vi "Car Wash System.vi"() -> ()   [LabVIEW 2024]
uses:
  ctl/Options Indicator.ctl
  ctl/Wash Options in.ctl
  ctl/State Machine.ctl
  ctl/Login State Machine.ctl
  <vilib>/Utility/file.llb/Write Delimited Spreadsheet (string).vi
  <vilib>/Utility/file.llb/Read Delimited Spreadsheet (string).vi
panel:
  in  "stop":bool
  in  "Options":T1
  in  "Start Button":bool
  out "Car Wash Indicator":T2
  out "Wash Vacant":bool
  out "Elapsed Time":dbl format="%#_3g"
  in  "Car Position Slider":u8(slide) max=3 scale=0.0..4.0
  in  "Stop Program":bool
  out "appended path":path
  out "Numeric":i32
  in  "Tab Control":enum32{"Login", "Register"}(tab)
  in  "Login":bool
  in  "Username":string
  in  "Password":string
  out "Status":bool
  in  "Username":string
  in  "Password":string
  in  "Register":bool
  out "Array":string[](array[string])
  out "error out":errorcluster
  in  "error in":errorcluster
  # "Entry Console"
  # "Car Wash Display"
  # "Wash Entry"
  # "Wash Options"
  # "Car Wash Indicator"
  # "Start"
  # "Car Position Simulation"
  # "Underbody Wash\nBug Remover"
  # "Pre-Soak\nH-P Wash\nL-P Wax\nSpot Free Rinse"
  # "Tire Shine\nAir Dry"
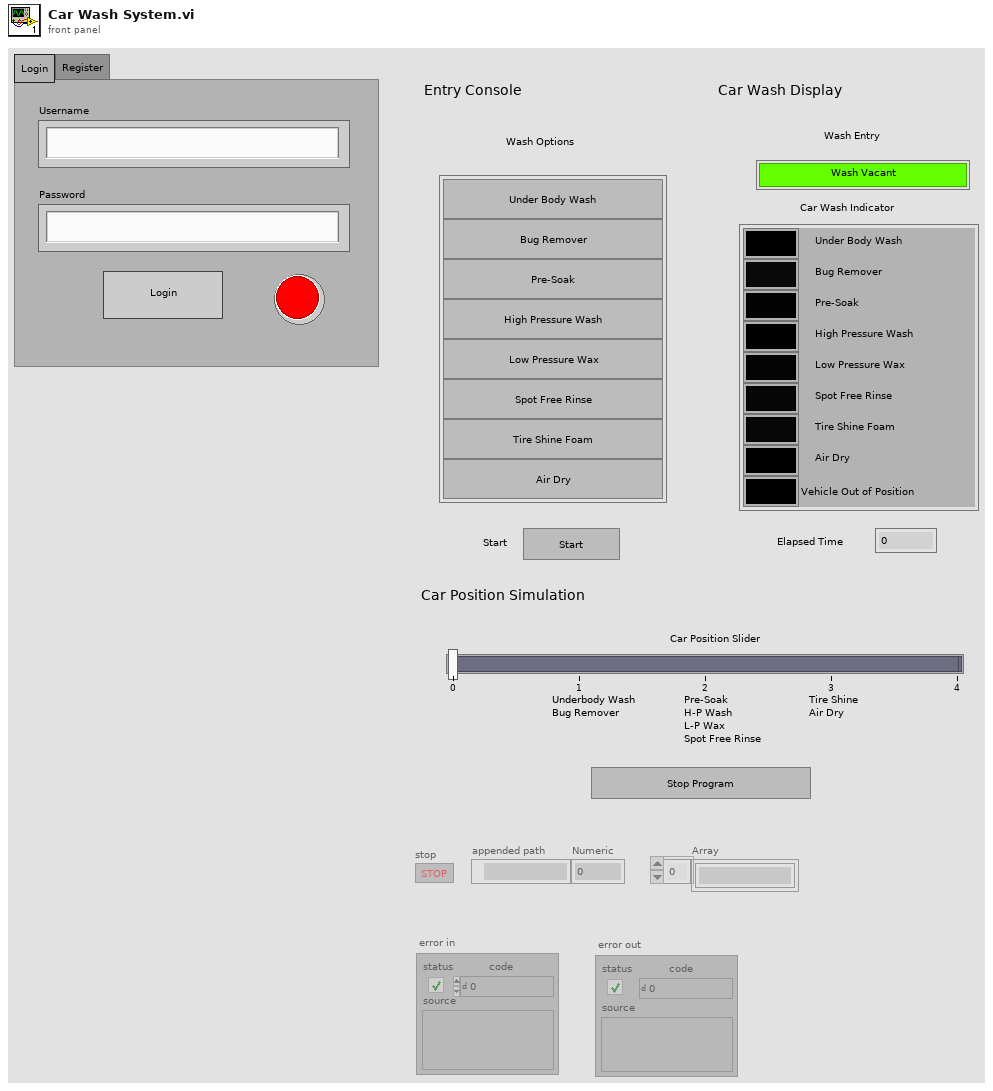
[diagram p1: front panel]
types:
  T1 = typedef "Wash Options in.ctl" = cluster{"Under Body Wash":bool, "Bug Remover":bool, "Pre-Soak":bool, "High Pressure Wash":bool, "Low Pressure Wax":bool, "Spot Free Rinse":bool, "Tire Shine Foam":bool, "Air Dry":bool}
  T2 = typedef "Options Indicator.ctl" = cluster{"Under Body Wash":bool, "Bug Remover":bool, "Pre-Soak":bool, "High Pressure Wash":bool, "Low Pressure Wax":bool, "Spot Free Rinse":bool, "Tire Shine Foam":bool, "Air Dry":bool, "Vehicle Out of Position":bool}
  T3 = typedef "Login State Machine.ctl" = enum16{"Init", "Wait", "Check", "Login", "Registration", "End"}
  T4 = typedef "State Machine.ctl" = enum16{"Initialize", "Wait", "Start", "Time", "Reset", "Stop"}
  T5 = enum8{"Enabled", "Disabled", "Disabled and Grayed Out"}
  T6 = cluster{"Under Body Wash":bool, "Bug Remover":bool, "Pre-Soak":bool, "High Pressure Wash":bool, "Low Pressure Wax":bool, "Spot Free Rinse":bool, "Tire Shine Foam":bool, "Air Dry":bool, "Vehicle Out of Position":bool}
  T7 = typedef "WashOptionsTypedef.ctl" = enum16{"Under Body Wash", "Bug Remover", "Pre-soak", "High Pressure Wash", "Low Pressure Wash", "Spot Free Rinse", "Tire Shine Foam", "Air Dry"}
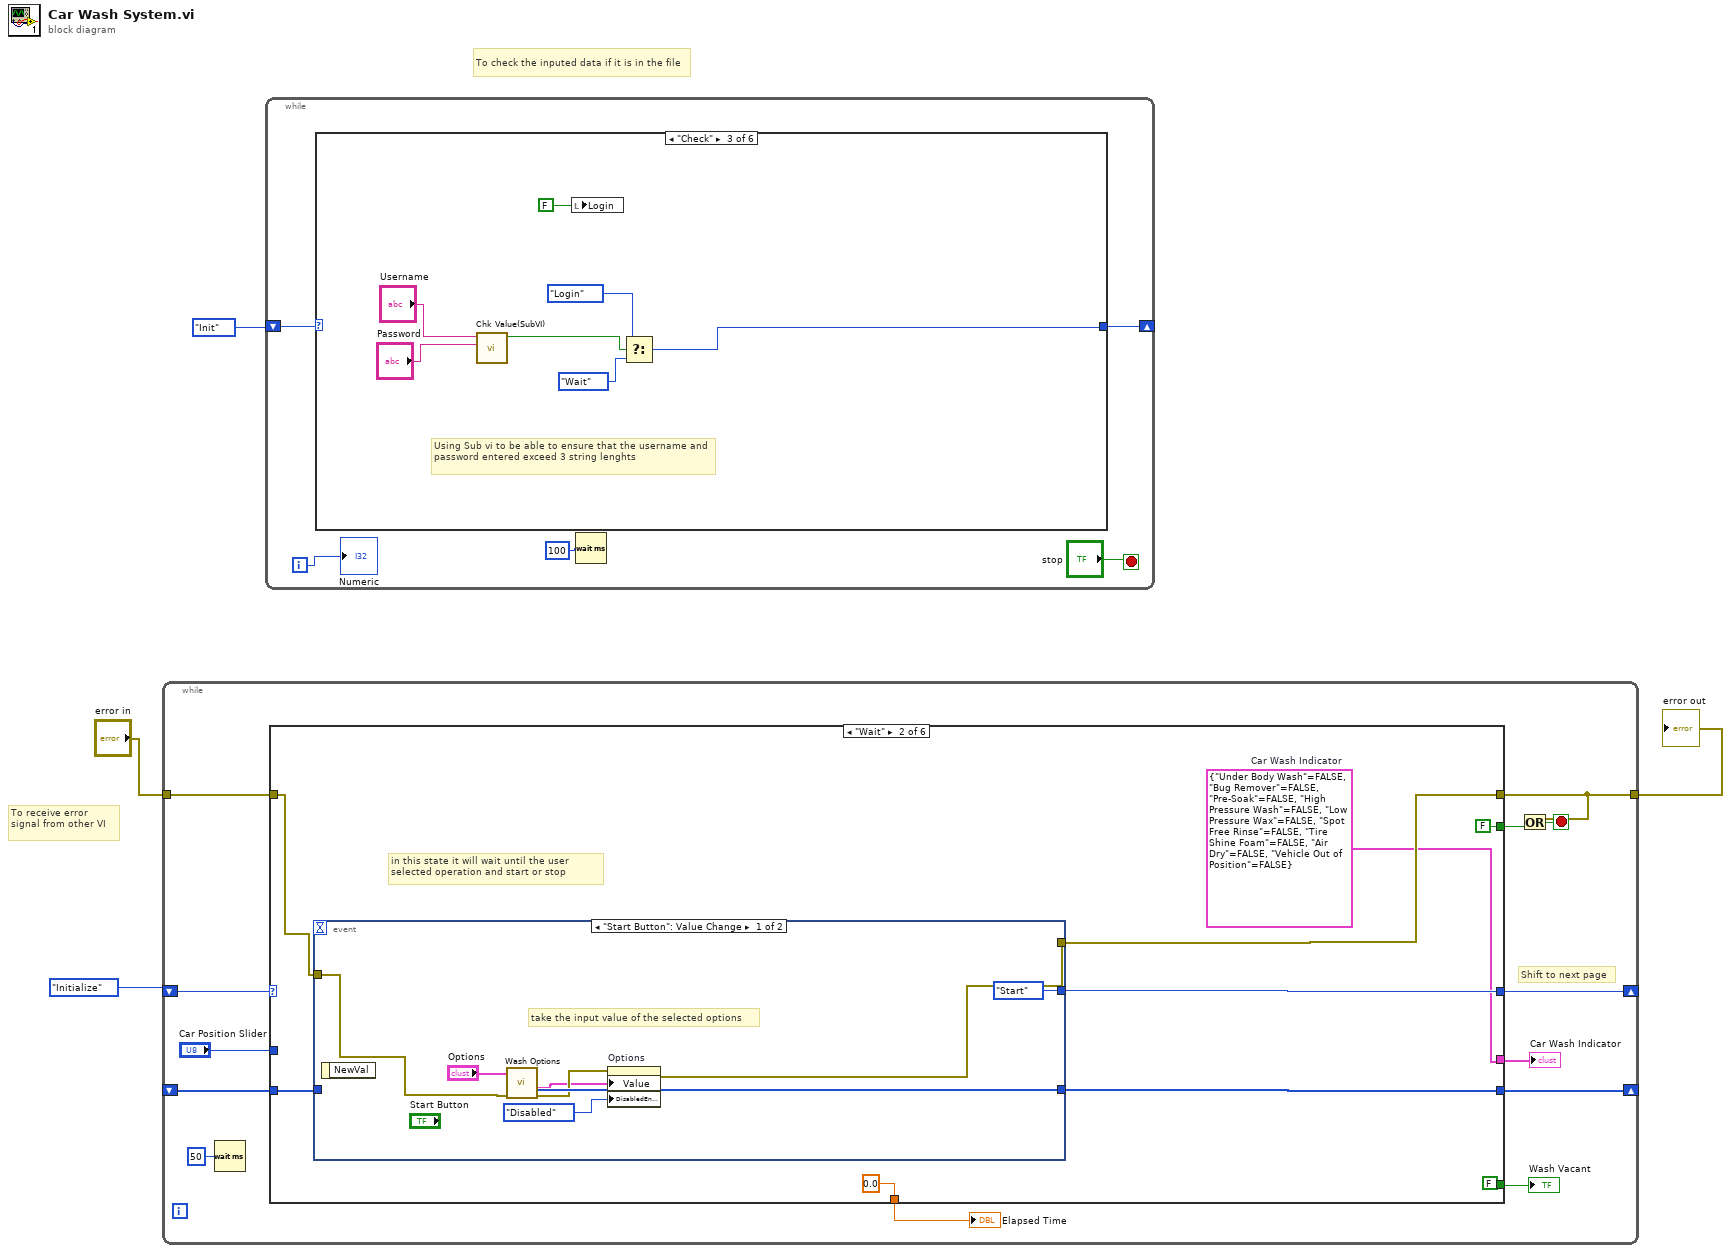
[diagram p0: block diagram]
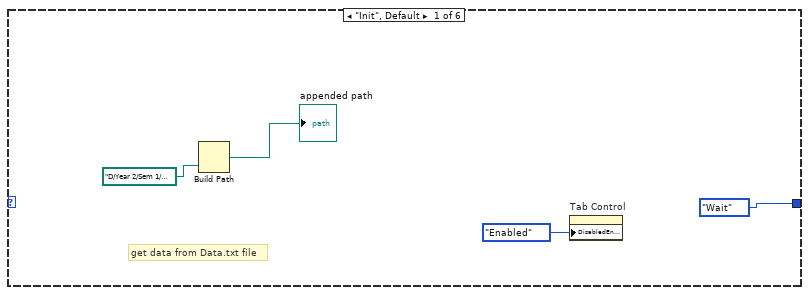
[diagram p2: hidden frame]
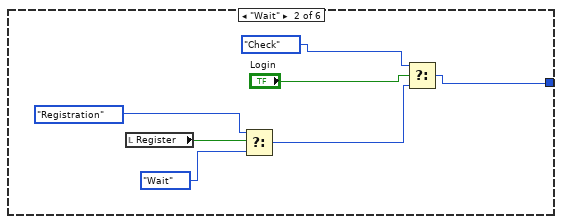
[diagram p3: hidden frame]
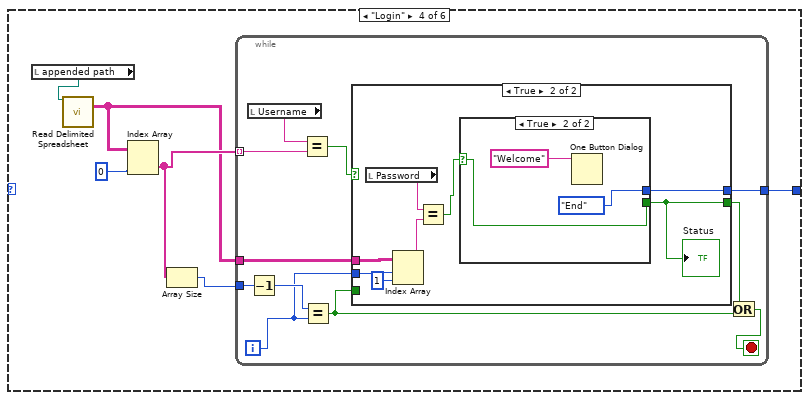
[diagram p4: hidden frame]
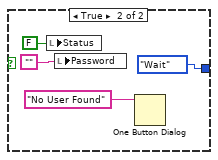
[diagram p6: hidden frame]
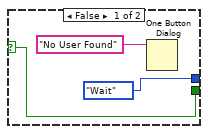
[diagram p7: hidden frame]
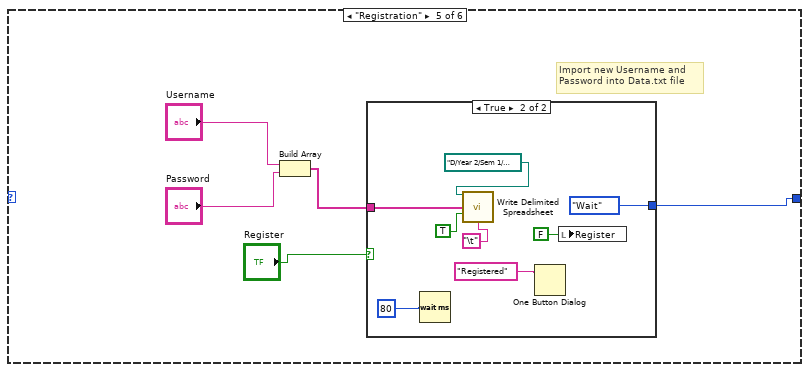
[diagram p8: hidden frame]
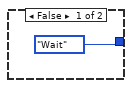
[diagram p9: hidden frame]
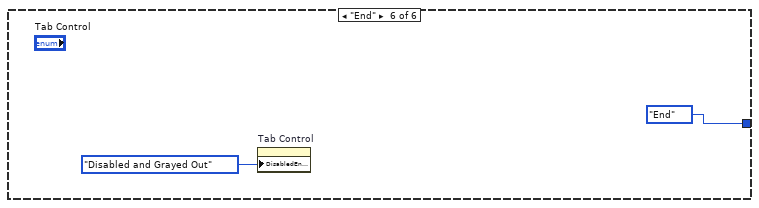
[diagram p10: hidden frame]
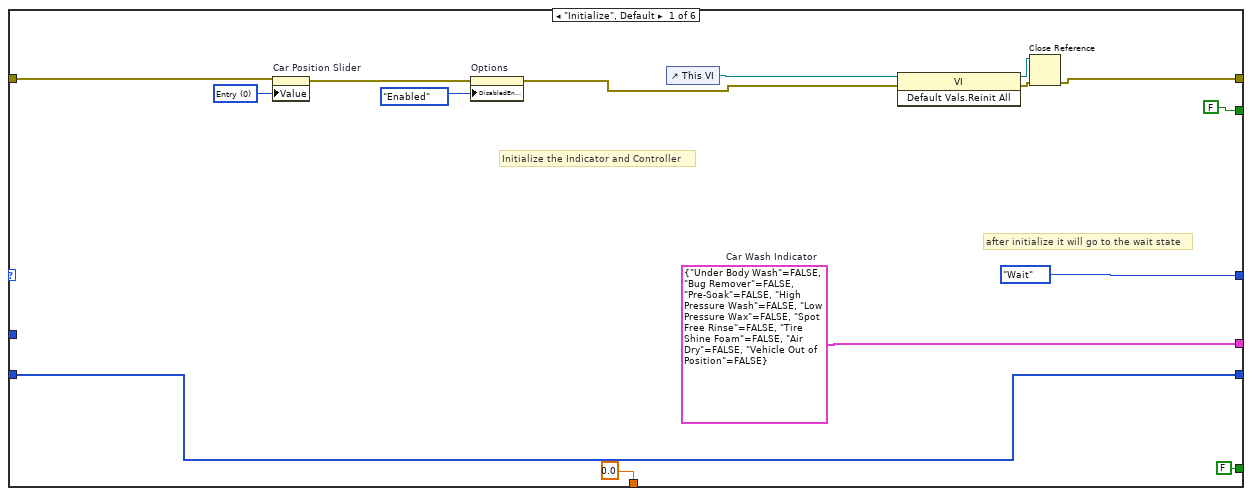
[diagram p11: hidden frame]
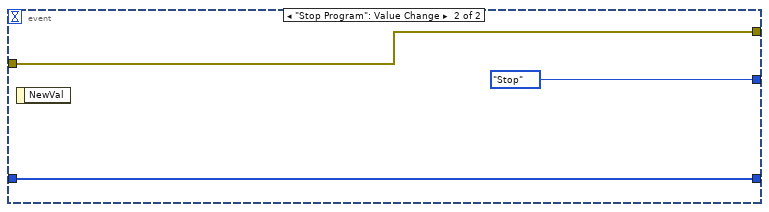
[diagram p12: hidden frame]
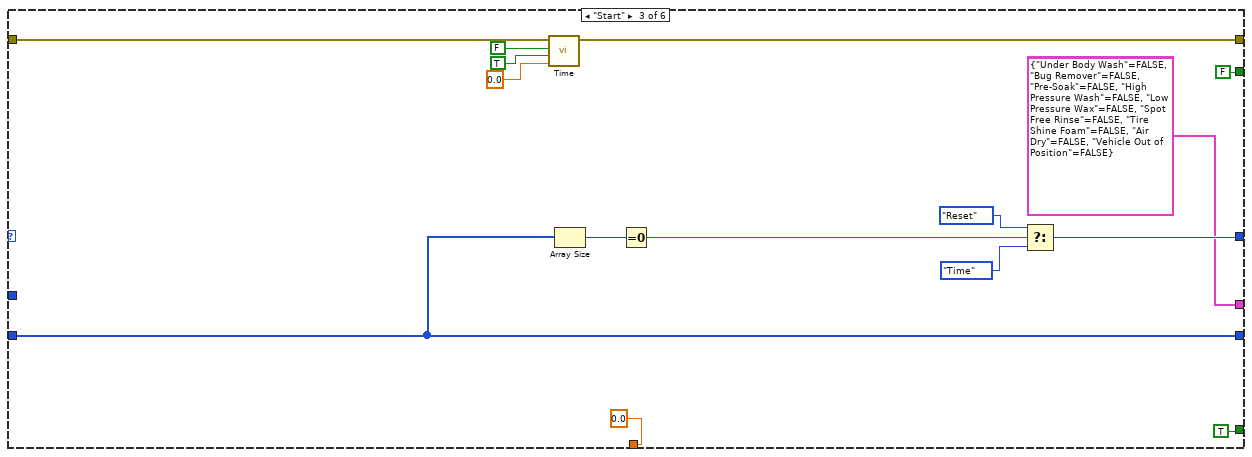
[diagram p13: hidden frame]
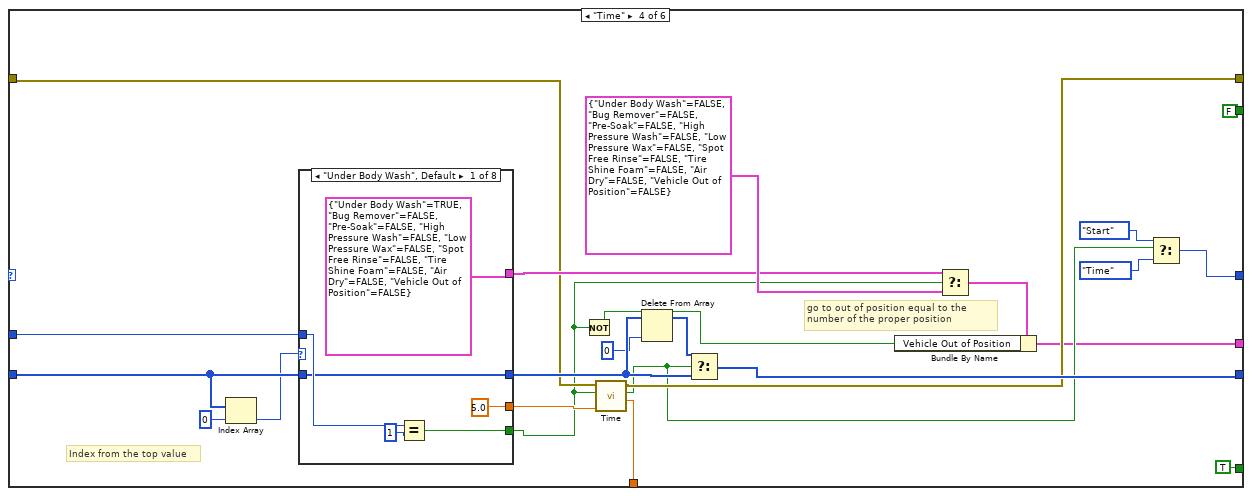
[diagram p14: hidden frame]
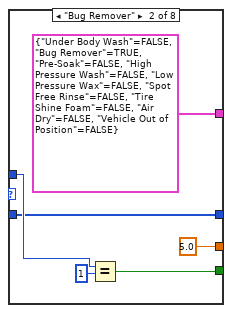
[diagram p15: hidden frame]
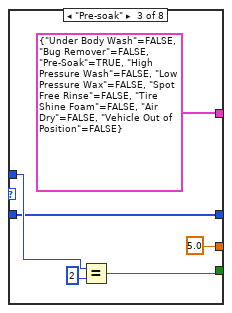
[diagram p16: hidden frame]
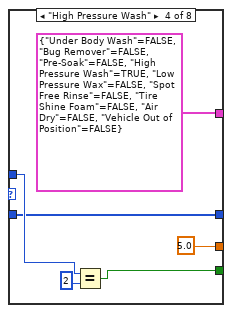
[diagram p17: hidden frame]
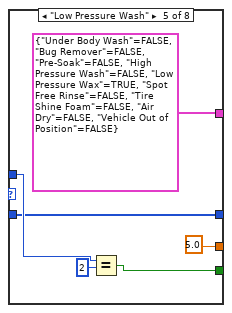
[diagram p18: hidden frame]
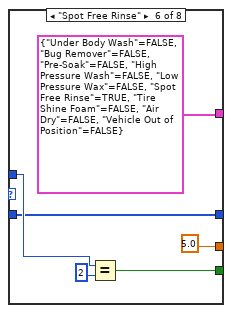
[diagram p19: hidden frame]
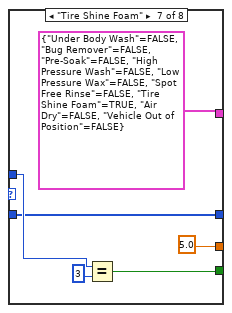
[diagram p20: hidden frame]
diagram:
  # "To check the inputed data if it is in the file"
  # "To receive error signal from other VI"
  n1 = while {
    shift-right: [w15] -> _
    shift-left: State_Machine."Initialize" -> [w16]
    shift-right: [w14] -> _
    shift-left: _ -> [w13]
    tunnel: "error in" -> [w11]
    tunnel: [w9] -> w4
    stop <- w10 stop-if-true
    # "Shift to next page"
    n2 = Wait (ms)(milliseconds to wait=u32 50) -> ()  [unwired: 1 out]
    n3 = case shown="\"Wait\"" w16 {
      tunnel: "Car Position Slider" -> [_ _ _ w89 w149 _]
      tunnel: [State_Machine."Wait" w41 w65 w76 w146 w156] -> w15
      tunnel: [w31 w40 w62 w79 w145 w170] -> w14
      tunnel: w13 -> [w31 w39 w62 w91 w145 w170]
      tunnel: w11 -> [w25 w38 w61 w75 w144 w165]
      tunnel: [w27 w37 w60 w74 w144 w164] -> w9
      tunnel: [FALSE FALSE FALSE FALSE FALSE TRUE] -> w8
      tunnel: [0.0 ("Elapsed Time") 0.0 ("Elapsed Time") 0.0 ("Elapsed Time") w70 0.0 ("Elapsed Time") 0.0 ("Elapsed Time")] -> w7
      tunnel: [FALSE ("Wash Vacant") FALSE ("Wash Vacant") TRUE ("Wash Vacant") TRUE ("Wash Vacant") TRUE ("Wash Vacant") FALSE ("Wash Vacant")] -> w6
      tunnel: [w18 w33 T6 {"Under Body Wash"=FALSE, "Bug Remover"=FALSE, "Pre-Soak"=FALSE, "High Pressure Wash"=FALSE, "Low Pressure Wax"=FALSE, "Spot Free Rinse"=FALSE, "Tire Shine Foam"=FALSE, "Air Dry"=FALSE, "Vehicle Out of Position"=FALSE} ("Car Wash Indicator") w68 w140 w157] -> w5
      frame "Initialize", Default {
        w26 = u8 0 items=["Entry", "Station 1", "Station 2", "Station 3", "Exit"] ("Car Position Slider")
        w18 = T6 {"Under Body Wash"=FALSE, "Bug Remover"=FALSE, "Pre-Soak"=FALSE, "High Pressure Wash"=FALSE, "Low Pressure Wax"=FALSE, "Spot Free Rinse"=FALSE, "Tire Shine Foam"=FALSE, "Air Dry"=FALSE, "Vehicle Out of Position"=FALSE}  # Car Wash Indicator
        # "after initialize it will go to the wait state"
        # "Initialize the Indicator and Controller"
        n4 = property on="Car Position Slider" class="Slide (strict)"(error in=w25, "Value"=w26) -> (error out=w23:errorcluster)  [unwired: 1 in, 1 out]
        n5 = property on="Options" class="Clust (strict)"(error in=w23, "DisabledEnum"=T5."Enabled" ("Disabled")) -> (error out=w22:errorcluster)  [unwired: 1 in, 1 out]
        n6 = control-ref of="This VI"() -> (w30:refnum<vi>)
        n7 = invoke class="VI" method="Default Vals.Reinit All"(reference=w30, error in=w22) -> (reference out=w28:refnum<vi>, error out=w29:errorcluster)  [unwired: 1 in, 1 out]
        n8 = Close Reference(reference=w28, error in (no error)=w29) -> (error out=w27:errorcluster)
      }
      frame "Wait" {
        w33 = T6 {"Under Body Wash"=FALSE, "Bug Remover"=FALSE, "Pre-Soak"=FALSE, "High Pressure Wash"=FALSE, "Low Pressure Wax"=FALSE, "Spot Free Rinse"=FALSE, "Tire Shine Foam"=FALSE, "Air Dry"=FALSE, "Vehicle Out of Position"=FALSE}  # Car Wash Indicator
        # "in this state it will wait until the user selected operation and start or stop"
        n9 = event shown="[0] \"Start Button\": Value Change" {
          selector: _ -> [_ _]
          dyn-events: _ -> [_ _]
          timeout: _ -> [_ _]
          tunnel: [State_Machine."Start" State_Machine."Stop"] -> w41
          tunnel: [w48 w51] -> w40
          tunnel: w39 -> [_ w51]
          tunnel: w38 -> [w45 w50]
          tunnel: [w43 w50] -> w37
          event "Start Button": Value Change {
            # "take the input value of the selected options"
            n10 = event-data() -> ()  [unwired: 1 in, 1 out]
            n11 = call "Wash Options.vi"("error in"=w45, "input"="Options") -> ("error out"=w44:errorcluster, "output"=w42:T1, "Array"=w48:T7[])  [unwired: 7 in]
            n12 = property on="Options" class="Clust (strict)"(error in=w44, "Value"=w42, "DisabledEnum"=T5."Disabled" ("Disabled")) -> (error out=w43:errorcluster)  [unwired: 1 in, 1 out]
          }
          event "Stop Program": Value Change {
            n13 = event-data() -> ()  [unwired: 1 in, 1 out]
          }
        }
      }
      frame "Start" {
        (unwired) T6 {"Under Body Wash"=FALSE, "Bug Remover"=FALSE, "Pre-Soak"=FALSE, "High Pressure Wash"=FALSE, "Low Pressure Wax"=FALSE, "Spot Free Rinse"=FALSE, "Tire Shine Foam"=FALSE, "Air Dry"=FALSE, "Vehicle Out of Position"=FALSE} ("Car Wash Indicator")
        n14 = call "Time.vi"("Wished Time"=0.0, "Reset"=TRUE, "Advance Time"=FALSE, "error in"=w61) -> ("error out"=w60:errorcluster)  [unwired: 5 in, 2 out]
        n15 = Array Size(array=w62) -> (size(s)=w64:i32)
        n16 = Equal To 0?(x=w64) -> (x = 0?=w63:bool)
        n17 = Select(t=State_Machine."Reset", s=w63, f=State_Machine."Time") -> (s? t:f=w65:T4)
      }
      frame "Time" {
        # "go to out of position equal to the number of the proper position"
        # "Index from the top value"
        n18 = Index Array "Index Array"(array=w91, index=0) -> (element=w90:T7)
        n19 = case shown="\"Under Body Wash\", Default" w90 {
          tunnel: w91 -> [w94 w100 w106 w112 w119 w124 w130 w136]
          tunnel: w89 -> [w97 w102 w109 w114 w121 w126 w132 w138]
          tunnel: [w95 w101 w107 w113 w120 w125 w131 w137] -> w73
          tunnel: [w94 w100 w106 w112 w119 w124 w130 w136] -> w81
          tunnel: [5.0 5.0 5.0 5.0 5.0 5.0 5.0 5.0] -> w88
          tunnel: [T6 {"Under Body Wash"=TRUE, "Bug Remover"=FALSE, "Pre-Soak"=FALSE, "High Pressure Wash"=FALSE, "Low Pressure Wax"=FALSE, "Spot Free Rinse"=FALSE, "Tire Shine Foam"=FALSE, "Air Dry"=FALSE, "Vehicle Out of Position"=FALSE} ("Car Wash Indicator") T6 {"Under Body Wash"=FALSE, "Bug Remover"=TRUE, "Pre-Soak"=FALSE, "High Pressure Wash"=FALSE, "Low Pressure Wax"=FALSE, "Spot Free Rinse"=FALSE, "Tire Shine Foam"=FALSE, "Air Dry"=FALSE, "Vehicle Out of Position"=FALSE} ("Car Wash Indicator") T6 {"Under Body Wash"=FALSE, "Bug Remover"=FALSE, "Pre-Soak"=TRUE, "High Pressure Wash"=FALSE, "Low Pressure Wax"=FALSE, "Spot Free Rinse"=FALSE, "Tire Shine Foam"=FALSE, "Air Dry"=FALSE, "Vehicle Out of Position"=FALSE} ("Car Wash Indicator") T6 {"Under Body Wash"=FALSE, "Bug Remover"=FALSE, "Pre-Soak"=FALSE, "High Pressure Wash"=TRUE, "Low Pressure Wax"=FALSE, "Spot Free Rinse"=FALSE, "Tire Shine Foam"=FALSE, "Air Dry"=FALSE, "Vehicle Out of Position"=FALSE} ("Car Wash Indicator") T6 {"Under Body Wash"=FALSE, "Bug Remover"=FALSE, "Pre-Soak"=FALSE, "High Pressure Wash"=FALSE, "Low Pressure Wax"=TRUE, "Spot Free Rinse"=FALSE, "Tire Shine Foam"=FALSE, "Air Dry"=FALSE, "Vehicle Out of Position"=FALSE} ("Car Wash Indicator") T6 {"Under Body Wash"=FALSE, "Bug Remover"=FALSE, "Pre-Soak"=FALSE, "High Pressure Wash"=FALSE, "Low Pressure Wax"=FALSE, "Spot Free Rinse"=TRUE, "Tire Shine Foam"=FALSE, "Air Dry"=FALSE, "Vehicle Out of Position"=FALSE} ("Car Wash Indicator") T6 {"Under Body Wash"=FALSE, "Bug Remover"=FALSE, "Pre-Soak"=FALSE, "High Pressure Wash"=FALSE, "Low Pressure Wax"=FALSE, "Spot Free Rinse"=FALSE, "Tire Shine Foam"=TRUE, "Air Dry"=FALSE, "Vehicle Out of Position"=FALSE} ("Car Wash Indicator") T6 {"Under Body Wash"=FALSE, "Bug Remover"=FALSE, "Pre-Soak"=FALSE, "High Pressure Wash"=FALSE, "Low Pressure Wax"=FALSE, "Spot Free Rinse"=FALSE, "Tire Shine Foam"=FALSE, "Air Dry"=TRUE, "Vehicle Out of Position"=FALSE} ("Car Wash Indicator")] -> w86
          frame "Under Body Wash", Default {
            n20 = Equal?(x=w97, y=u8 1) -> (x = y?=w95:bool)
          }
          frame "Bug Remover" {
            n21 = Equal?(x=w102, y=u8 1) -> (x = y?=w101:bool)
          }
          frame "Pre-soak" {
            n22 = Equal?(x=w109, y=u8 2) -> (x = y?=w107:bool)
          }
          frame "High Pressure Wash" {
            n23 = Equal?(x=w114, y=u8 2) -> (x = y?=w113:bool)
          }
          frame "Low Pressure Wash" {
            n24 = Equal?(x=w121, y=u8 2) -> (x = y?=w120:bool)
          }
          frame "Spot Free Rinse" {
            n25 = Equal?(x=w126, y=u8 2) -> (x = y?=w125:bool)
          }
          frame "Tire Shine Foam" {
            n26 = Equal?(x=w132, y=u8 3) -> (x = y?=w131:bool)
          }
          frame "Air Dry" {
            n27 = Equal?(x=w138, y=u8 3) -> (x = y?=w137:bool)
          }
        }
        n28 = Not(x=w73) -> (.not. x?=w84:bool)
        n29 = call "Time.vi"("Wished Time"=w88, "Advance Time"=w73, "error in"=w75) -> ("Elapsed Time"=w70:dbl, "Expired"=w72:bool, "error out"=w74:errorcluster)  [unwired: 6 in]
        n30 = Delete From Array "Delete From Array"(array=w81, index=0) -> (array with subset deleted=w82:T7[])  [unwired: 1 in, 1 out]
        n31 = Select(t=w82, s=w72, f=w81) -> (s? t:f=w79:T7[])
        n32 = Select(t=w86, s=w73, f=T6 {"Under Body Wash"=FALSE, "Bug Remover"=FALSE, "Pre-Soak"=FALSE, "High Pressure Wash"=FALSE, "Low Pressure Wax"=FALSE, "Spot Free Rinse"=FALSE, "Tire Shine Foam"=FALSE, "Air Dry"=FALSE, "Vehicle Out of Position"=FALSE} ("Car Wash Indicator")) -> (s? t:f=w85:T6)
        n33 = Bundle By Name(cluster=w85, "Vehicle Out of Position"=w84) -> (w68:T6)
        n34 = Select(t=State_Machine."Start", s=w72, f=State_Machine."Time") -> (s? t:f=w76:T4)
      }
      frame "Reset" {
        w140 = T6 {"Under Body Wash"=FALSE, "Bug Remover"=FALSE, "Pre-Soak"=FALSE, "High Pressure Wash"=FALSE, "Low Pressure Wax"=FALSE, "Spot Free Rinse"=FALSE, "Tire Shine Foam"=FALSE, "Air Dry"=FALSE, "Vehicle Out of Position"=TRUE}  # Car Wash Indicator
        (unwired) T6 {"Under Body Wash"=FALSE, "Bug Remover"=FALSE, "Pre-Soak"=FALSE, "High Pressure Wash"=FALSE, "Low Pressure Wax"=FALSE, "Spot Free Rinse"=FALSE, "Tire Shine Foam"=FALSE, "Air Dry"=FALSE, "Vehicle Out of Position"=FALSE} ("Car Wash Indicator")
        # "last car position 4, Exit. will initialize the indicator and controller"
        n35 = Equal?(x=w149, y=u8 4) -> (x = y?=w150:bool)
        n36 = Select(t=State_Machine."Initialize", s=w150, f=State_Machine."Reset") -> (s? t:f=w146:T4)
      }
      frame "Stop" {
        w166 = u8 0 items=["Entry", "Station 1", "Station 2", "Station 3", "Exit"] ("Car Position Slider")
        w157 = T6 {"Under Body Wash"=FALSE, "Bug Remover"=FALSE, "Pre-Soak"=FALSE, "High Pressure Wash"=FALSE, "Low Pressure Wax"=FALSE, "Spot Free Rinse"=FALSE, "Tire Shine Foam"=FALSE, "Air Dry"=FALSE, "Vehicle Out of Position"=FALSE}  # Car Wash Indicator
        (unwired) T6 {"Under Body Wash"=FALSE, "Bug Remover"=FALSE, "Pre-Soak"=FALSE, "High Pressure Wash"=FALSE, "Low Pressure Wax"=FALSE, "Spot Free Rinse"=FALSE, "Tire Shine Foam"=FALSE, "Air Dry"=FALSE, "Vehicle Out of Position"=FALSE} ("Car Wash Indicator")
        # "Reset everything into default"
        n37 = flat-sequence {
          tunnel: [w172] -> w152
          tunnel: w152 -> [w181]
          frame #0 {
            # "separator"
            n38 = for {
              N: 3 -> [_]
              tunnel: [w176] -> w173 mode=indexing
              i -> [w177]
              # "csv file header"
              n39 = case shown="2" w177 {
                tunnel: ["Date" "Time" "Selection"] -> w176
                frame 0, Default {
                }
                frame 1 {
                }
                frame 2 {
                }
              }
            }
            "Array" <- w173
            n40 = call-poly <vilib>:"Write Delimited Spreadsheet.vi"("file path (dialog if empty)"=path "D:/Year 2/Sem 1/SPCC/ASSIGNMENT/Car Wash Assignment/Txt/logging.txt", "1D data"=w173, "delimiter (\\t)"="\t") -> ("new file path (Not A Path if cancelled)"=w172:path)  [unwired: 11 in, 1 out]
          }
          frame #1 {
            n41 = while {
              tunnel: w181 -> [w185]
              stop <- FALSE stop-if-true
              n42 = for {
                N: 3 -> [_]
                tunnel: [w188] -> w183 mode=indexing
                i -> [w189]
                # "take the real time,date and options"
                n43 = case shown="0, Default" w189 {
                  tunnel: [w190 w191 w192] -> w188
                  frame 0, Default {
                    # "Date"
                    n44 = Get Date/Time String() -> (date string=w190:string)  [unwired: 3 in, 1 out]
                  }
                  frame 1 {
                    # "Time"
                    n45 = Get Date/Time String() -> (time string=w191:string)  [unwired: 3 in, 1 out]
                  }
                  frame 2 {
                    n46 = property on="Options" class="Clust (strict)"() -> ("Label.Text"=w193:string)  [unwired: 2 in, 2 out]
                    n47 = Concatenate Strings(w193) -> (w192:string)
                  }
                }
              }
              n48 = call-poly <vilib>:"Write Delimited Spreadsheet.vi"("file path (dialog if empty)"=w185, "1D data"=w183, "append to file? (new file:F)"=FALSE, "delimiter (\\t)"="\t") -> ()  [unwired: 10 in, 2 out]
            }
          }
        }
        n49 = property on="Car Position Slider" class="Slide (strict)"(error in=w165, "Value"=w166) -> (error out=w162:errorcluster)  [unwired: 1 in, 1 out]
        n50 = property on="Options" class="Clust (strict)"(error in=w162, "DisabledEnum"=T5."Enabled" ("Disabled")) -> (error out=w161:errorcluster)  [unwired: 1 in, 1 out]
        n51 = control-ref of="This VI"() -> (w169:refnum<vi>)
        n52 = invoke class="VI" method="Default Vals.Reinit All"(reference=w169, error in=w161) -> (reference out=w167:refnum<vi>, error out=w168:errorcluster)  [unwired: 1 in, 1 out]
        n53 = Close Reference(reference=w167, error in (no error)=w168) -> (error out=w164:errorcluster)
        n54 = Select(t=State_Machine."Stop", s="Stop Program", f=State_Machine."Stop") -> (s? t:f=w156:T4)
      }
    }
    "Elapsed Time" <- w7
    "Wash Vacant" <- w6
    "Car Wash Indicator" <- w5
    n55 = Or(x=w9, y=w8) -> (x .or. y?=w10:bool)
  }
  "error out" <- w4
  n56 = while {
    shift-right: [w195] -> _
    shift-left: Login_State_Machine."Init" -> [w196]
    i -> [w197]
    stop <- "stop" stop-if-true
    n57 = case shown="\"Check\"" w196 {
      tunnel: [Login_State_Machine."Wait" w209 w215 w217 w254 Login_State_Machine."End"] -> w195
      frame "Init", Default {
        # "get data from Data.txt file"
        n58 = Build Path(name or relative path=path "D:/Year 2/Sem 1/SPCC/ASSIGNMENT/Car Wash Assignment/Txt/Data.txt") -> (appended path=→"appended path":path)  [unwired: 1 in]
        n59 = property on="Tab Control" class="TabCtl (strict)"("DisabledEnum"=T5."Enabled" ("Disabled")) -> ()  [unwired: 2 in, 2 out]
      }
      frame "Wait" {
        n60 = local read "Register"() -> (w207:bool)
        n61 = Select(t=Login_State_Machine."Registration", s=w207, f=Login_State_Machine."Wait") -> (s? t:f=w205:T3)
        n62 = Select(t=Login_State_Machine."Check", s="Login", f=w205) -> (s? t:f=w209:T3)
      }
      frame "Check" {
        # "Using Sub vi to be able to ensure that the username and password entered exceed 3 string lenghts"
        n63 = call "Chk Value(SubVI).vi"("Password"="Password", "User Name"="Username") -> ("Boolean"=w216:bool)  [unwired: 9 in]
        n64 = local write "Login"(FALSE ("btnLogin")) -> ()
        n65 = Select(t=Login_State_Machine."Login", s=w216, f=Login_State_Machine."Wait") -> (s? t:f=w215:T3)
      }
      frame "Login" {
        n66 = local read "appended path"() -> (w222:path)
        n67 = call-poly <vilib>:"Read Delimited Spreadsheet.vi"("file path (dialog if empty)"=w222) -> ("all rows"=w219:string[][])  [unwired: 9 in, 5 out]
        n68 = Index Array(array=w219, index (col)=0) -> (element=w220:string[])  [unwired: 1 in]
        n69 = Array Size(array=w220) -> (size(s)=w218:i32)
        n70 = while {
          tunnel: w220 -> [w233] mode=indexing
          tunnel: w219 -> [w232]
          tunnel: w218 -> [w231]
          tunnel: [w223] -> w217
          i -> [w229]
          stop <- w228 stop-if-true
          n71 = local read "Username"() -> (w224:string)
          n72 = Decrement(x=w231) -> (x-1=w230:i32)
          n73 = Equal?(x=w224, y=w233) -> (x = y?=w225:bool)
          n74 = Equal?(x=w230, y=w229) -> (x = y?=w226:bool)
          n75 = case shown="True" w225 {
            tunnel: w232 -> [_ w247]
            tunnel: w229 -> [_ w245]
            tunnel: [_ w242] -> w227
            tunnel: w226 -> [w235 _]
            tunnel: [w234 w240] -> w223
            frame False {
              n76 = case shown="False" w235 {
                tunnel: [_ Login_State_Machine."Wait"] -> w234
                frame False {
                }
                frame True {
                  n77 = local write "Status"(FALSE ("Status")) -> ()
                  n78 = local write "Password"("") -> ()
                  n79 = One Button Dialog(message="No User Found") -> ()  [unwired: 1 in, 1 out]
                }
              }
            }
            frame True {
              n80 = local read "Password"() -> (w241:string)
              n81 = Index Array(array=w247, index (row)=w245, index (col)=1 ("disabled index (col)")) -> (element=w244:string)
              n82 = Equal?(x=w241, y=w244) -> (x = y?=w243:bool)
              n83 = case shown="True" w243 {
                selector: w243 -> [w250 w253]
                tunnel: [w250 w253] -> w242
                tunnel: [Login_State_Machine."Wait" Login_State_Machine."End"] -> w240
                frame False {
                  n84 = One Button Dialog(message="No User Found") -> ()  [unwired: 1 in, 1 out]
                }
                frame True {
                  n85 = One Button Dialog(message="Welcome") -> ()  [unwired: 1 in, 1 out]
                }
              }
              "Status" <- w242
            }
          }
          n86 = Or(x=w227, y=w226) -> (x .or. y?=w228:bool)
        }
      }
      frame "Registration" {
        # "Import new Username and Password into Data.txt file"
        n87 = Build Array("Username", "Password") -> (w256:string[])
        n88 = case shown="True" "Register" {
          tunnel: w256 -> [_ w266]
          tunnel: [Login_State_Machine."Wait" Login_State_Machine."Wait"] -> w254
          frame False {
          }
          frame True {
            n89 = Wait (ms)(milliseconds to wait=u32 80) -> ()  [unwired: 1 out]
            n90 = call-poly <vilib>:"Write Delimited Spreadsheet.vi"("file path (dialog if empty)"=path "D:/Year 2/Sem 1/SPCC/ASSIGNMENT/Car Wash Assignment/Txt/Data.txt" ("name or relative path"), "1D data"=w266, "append to file? (new file:F)"=TRUE, "delimiter (\\t)"="\t") -> ()  [unwired: 10 in, 2 out]
            n91 = One Button Dialog(message="Registered") -> ()  [unwired: 1 in, 1 out]
            n92 = local write "Register"(FALSE ("Register")) -> ()
          }
        }
      }
      frame "End" {
        n93 = property on="Tab Control" class="TabCtl (strict)"("DisabledEnum"=T5."Disabled and Grayed Out" ("Disabled")) -> ()  [unwired: 2 in, 2 out]
      }
    }
    n94 = Wait (ms)(milliseconds to wait=u32 100) -> ()  [unwired: 1 out]
    "Numeric" <- w197
  }
